vi "Get SC from raw signal.vi"(9 "Sampling Rate":dbl, 11 "raw SC":dbl[](array[numeric])) -> (3 "SC":dbl[](array[numeric]))   [LabVIEW 2014]
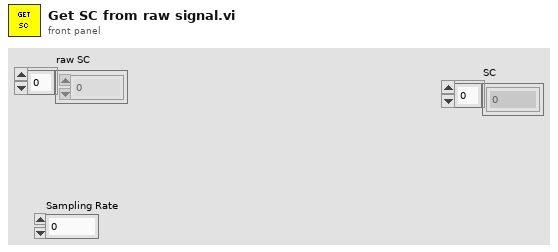
[diagram p1: front panel]
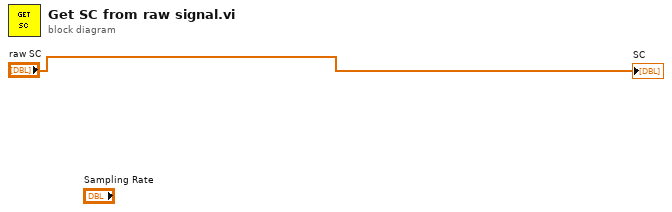
[diagram p0: block diagram]
diagram:
  "SC" <- "raw SC"
